vi "WILT Step Pause Dryer.vi"(7 "Station Number in":u32, 8 "Error In":errorcluster, 10 "Step 3 Input":T1, 11 "Dryer Step Pause In":T3 {"Night Cycle Count" format="%04d"; "Day Cycle Count" format="%04d"}) -> (0 "Error Out":errorcluster, 2 "Step 5 Output":T1, 3 "Dryer Step Pause Output":T3 {"Night Cycle Count" format="%04d"; "Day Cycle Count" format="%04d"})   [LabVIEW 2016]
uses:
  Type Definitions/WILT Station Test State Cluster.ctl
  Type Definitions/WILT Dryer Test State.ctl
  Type Definitions/WILT Dryer.ctl
  Type Definitions/WILT Dryer Details.ctl
  Type Definitions/WILT Agilent Channel Definition.ctl
  Type Definitions/WILT DAQ Data.ctl
  Globals/WILT Globals Main Program.vi
panel:
  # "Day"
  # "Night"
  # "Day"
  # "Night"
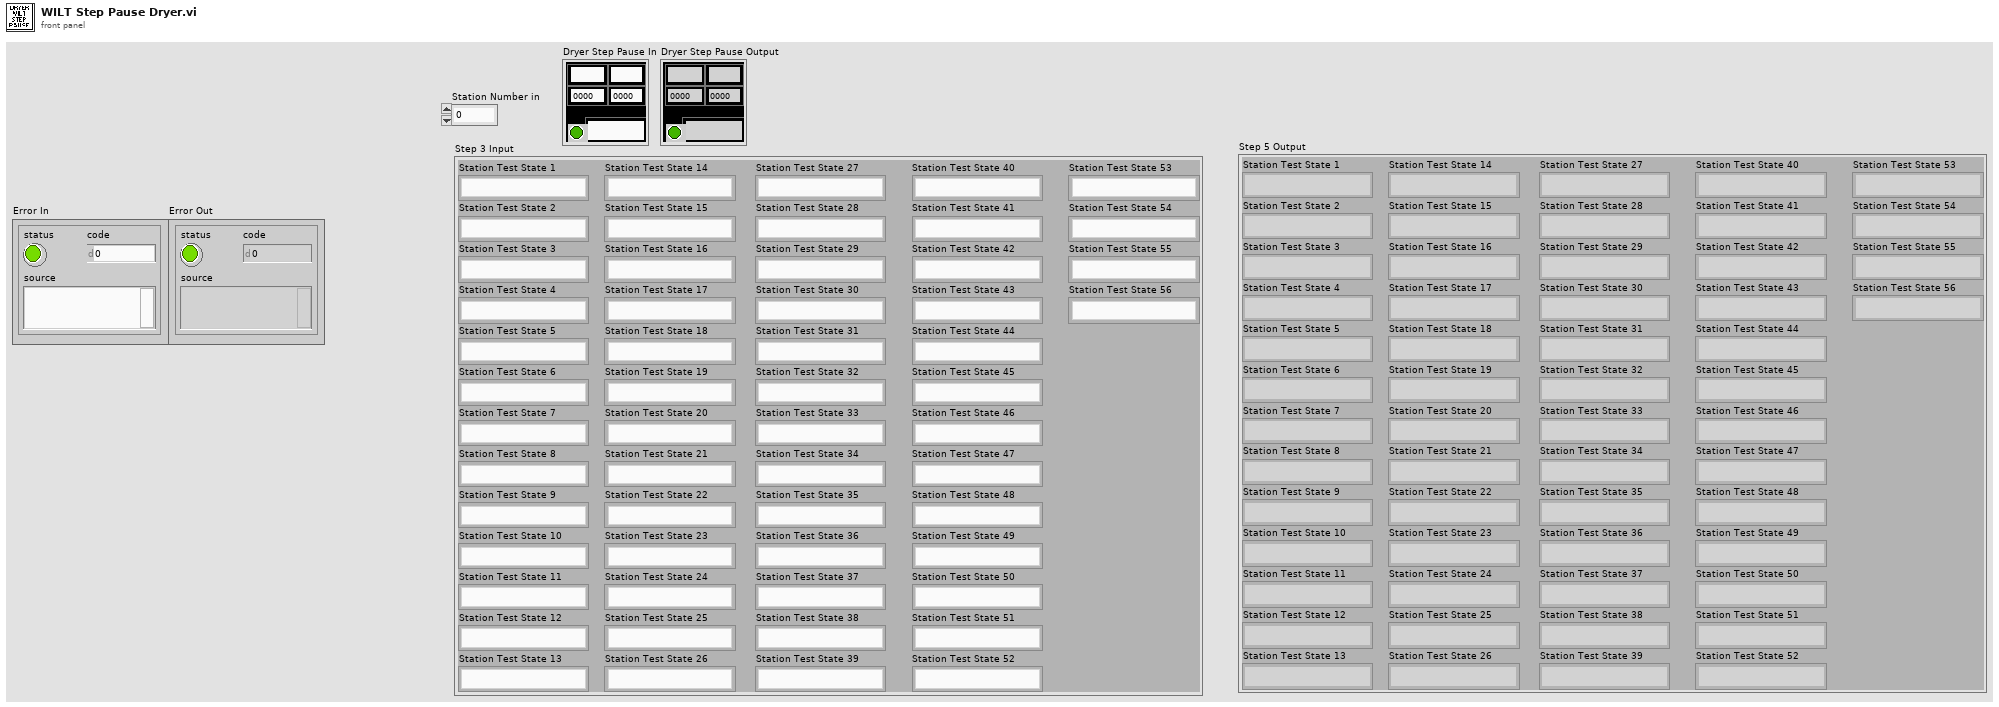
[diagram p1: front panel]
types:
  T1 = typedef "WILT Station Test State Cluster.ctl" = cluster{"Station Test State 1":T2, "Station Test State 2":T2, "Station Test State 3":T2, "Station Test State 4":T2, "Station Test State 5":T2, "Station Test State 6":T2, "Station Test State 7":T2, "Station Test State 8":T2, "Station Test State 9":T2, "Station Test State 10":T2, "Station Test State 11":T2, "Station Test State 12":T2, "Station Test State 13":T2, "Station Test State 14":T2, "Station Test State 15":T2, "Station Test State 16":T2, "Station Test State 17":T2, "Station Test State 18":T2, "Station Test State 19":T2, "Station Test State 20":T2, "Station Test State 21":T2, "Station Test State 22":T2, "Station Test State 23":T2, "Station Test State 24":T2, "Station Test State 25":T2, "Station Test State 26":T2, "Station Test State 27":T2, "Station Test State 28":T2, "Station Test State 29":T2, "Station Test State 30":T2, "Station Test State 31":T2, "Station Test State 32":T2, "Station Test State 33":T2, "Station Test State 34":T2, "Station Test State 35":T2, "Station Test State 36":T2, "Station Test State 37":T2, "Station Test State 38":T2, "Station Test State 39":T2, "Station Test State 40":T2, "Station Test State 41":T2, "Station Test State 42":T2, "Station Test State 43":T2, "Station Test State 44":T2, "Station Test State 45":T2, "Station Test State 46":T2, "Station Test State 47":T2, "Station Test State 48":T2, "Station Test State 49":T2, "Station Test State 50":T2, "Station Test State 51":T2, "Station Test State 52":T2, "Station Test State 53":T2, "Station Test State 54":T2, "Station Test State 55":T2, "Station Test State 56":T2}
  T2 = typedef "WILT Dryer Test State.ctl" = enum16{"No Serial Number", "Waiting for Dryer To Start", "Drying Clothes", "Water Injection 1 (On)", "Water Injection 1 Timer", "Water Injection 1 (Off)", "Pause Dryer", "Sending Start Stop CMD", "Pause Dryer 2", "Sending Start Stop CMD 2", "Drying Clothes 2", "Water Injection 2 (On)", "Water Injection 2 Timer", "Water Injection 2 (Off)", "Drying Clothes 3", "Cooling Down", "Sending Start Stop CMD 3", "Increment Cycle"}
  T3 = typedef "WILT Dryer.ctl" = cluster{"Lab ID":string, "Day Cycle Count":i32, "Station Label":string, "Dryer Details":T4, "Status Color":u32, "Invisible Button":bool, "Night Cycle Count":i32, "Station Index":i32, "Cycle Index":string, "Audit Alert":bool, "Agilent Channel Definition":T5, "DAQ Data":T6}
  T4 = typedef "WILT Dryer Details.ctl" = cluster{"Station":string, "Lab ID":string, "TR Number":string}
  T5 = typedef "WILT Agilent Channel Definition.ctl" = cluster{"Channel":string, "Station":string, "Label":string, "Agilent Station":string, "Data":dbl}
  T6 = typedef "WILT DAQ Data.ctl" = cluster{"L1 Current":dbl, "L2 Current":dbl, "Temperature  Deg F (TC)":dbl, "Volts":dbl, "Volts (208)":dbl, "SW (208)":dbl}
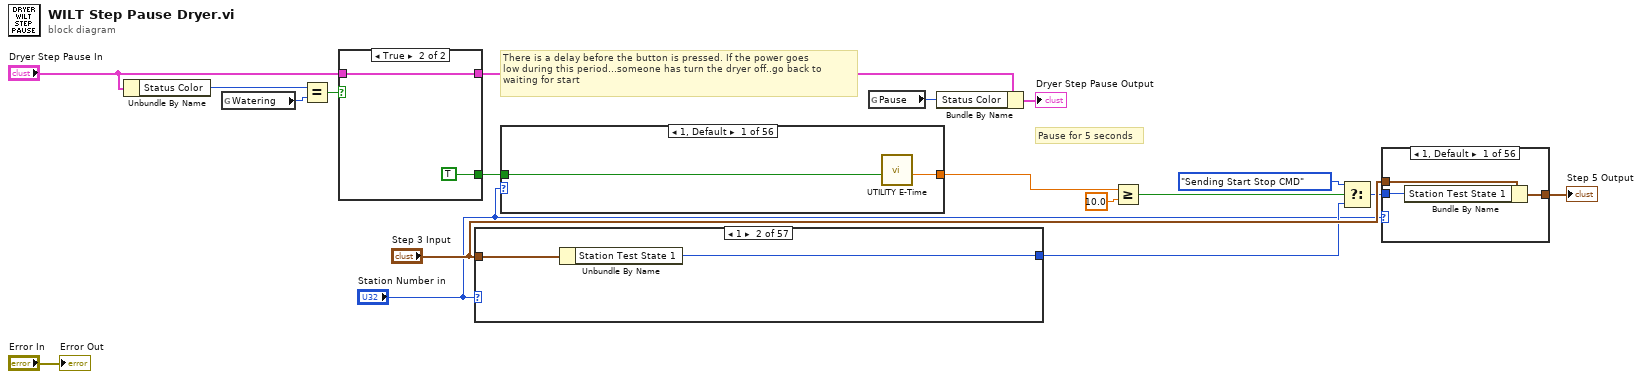
[diagram p0: block diagram]
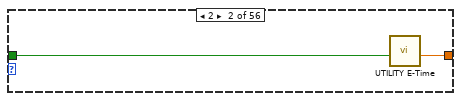
[diagram p2: hidden frame]
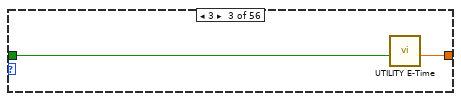
[diagram p3: hidden frame]
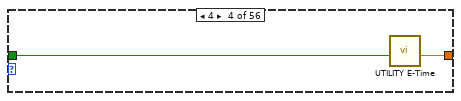
[diagram p4: hidden frame]
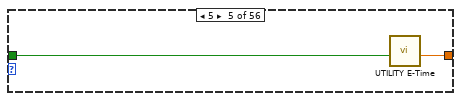
[diagram p5: hidden frame]
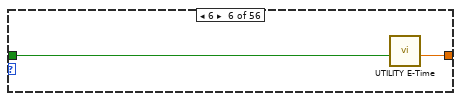
[diagram p6: hidden frame]
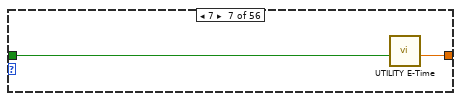
[diagram p7: hidden frame]
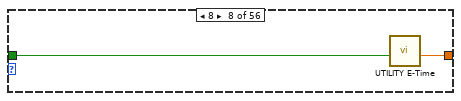
[diagram p8: hidden frame]
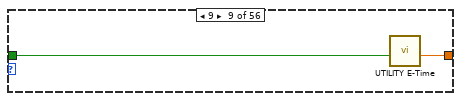
[diagram p9: hidden frame]
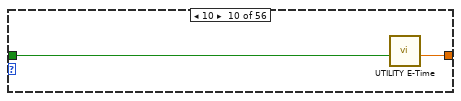
[diagram p10: hidden frame]
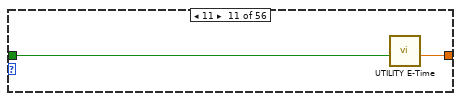
[diagram p11: hidden frame]
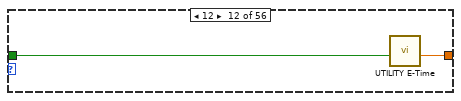
[diagram p12: hidden frame]
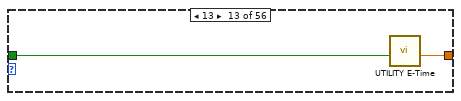
[diagram p13: hidden frame]
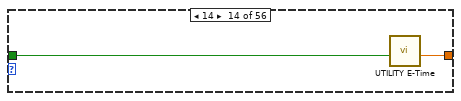
[diagram p14: hidden frame]
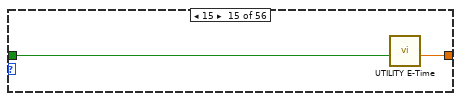
[diagram p15: hidden frame]
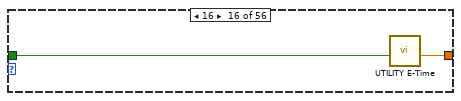
[diagram p16: hidden frame]
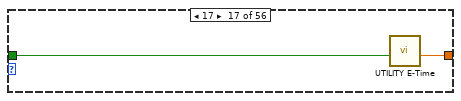
[diagram p17: hidden frame]
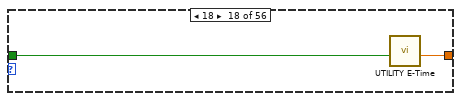
[diagram p18: hidden frame]
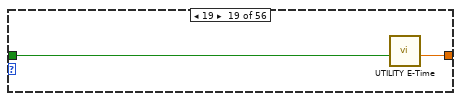
[diagram p19: hidden frame]
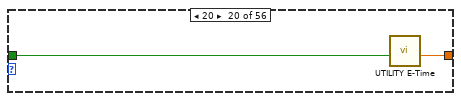
[diagram p20: hidden frame]
diagram:
  # "Pause for 5 seconds"
  # "There is a delay before the button is pressed. If the power goes\nlow during this period...someone has turn the dryer off..go back to \nwaiting for start"
  n1 = Unbundle By Name("Dryer Step Pause In") -> ("Status Color"=w12:u32)
  n2 = global read "WILT Globals Main Program.vi" "Watering"() -> (w4:u32)
  n3 = Equal?(x=w12, y=w4) -> (x = y?=w5:bool)
  n4 = case shown="True" w5 {
    tunnel: [FALSE TRUE] -> w3
    tunnel: "Dryer Step Pause In" -> [w19 w21]
    tunnel: [w19 w21] -> w2
    frame False {
    }
    frame True {
    }
  }
  n5 = case shown="1" "Station Number in" {
    tunnel: "Step 3 Input" -> [_ w25 w27 w29 w31 w33 w35 w37 w39 w41 w43 w45 w47 w49 w51 w53 w55 w57 w59 w61 w63 w65 w67 w69 w71 w73 w75 w77 w79 w81 w83 w85 w87 w89 w91 w93 w95 w97 w99 w101 w103 w105 w107 w109 w111 w113 w115 w117 w119 w121 w123 w125 w127 w129 w131 w133 w135]
    tunnel: [WILT_Dryer_Test_State."No Serial Number" ("Station Test State 56") w24 w26 w28 w30 w32 w34 w36 w38 w40 w42 w44 w46 w48 w50 w52 w54 w56 w58 w60 w62 w64 w66 w68 w70 w72 w74 w76 w78 w80 w82 w84 w86 w88 w90 w92 w94 w96 w98 w100 w102 w104 w106 w108 w110 w112 w114 w116 w118 w120 w122 w124 w126 w128 w130 w132 w134] -> w14
    frame 0, Default {
      # "This is not a station.\nDo nothing"
    }
    frame 1 {
      n6 = Unbundle By Name(w25) -> ("Station Test State 1"=w24:T2)
    }
    frame 2 {
      n7 = Unbundle By Name(w27) -> ("Station Test State 2"=w26:T2)
    }
    frame 3 {
      n8 = Unbundle By Name(w29) -> ("Station Test State 3"=w28:T2)
    }
    frame 4 {
      n9 = Unbundle By Name(w31) -> ("Station Test State 4"=w30:T2)
    }
    frame 5 {
      n10 = Unbundle By Name(w33) -> ("Station Test State 5"=w32:T2)
    }
    frame 6 {
      n11 = Unbundle By Name(w35) -> ("Station Test State 6"=w34:T2)
    }
    frame 7 {
      n12 = Unbundle By Name(w37) -> ("Station Test State 7"=w36:T2)
    }
    frame 8 {
      n13 = Unbundle By Name(w39) -> ("Station Test State 8"=w38:T2)
    }
    frame 9 {
      n14 = Unbundle By Name(w41) -> ("Station Test State 9"=w40:T2)
    }
    frame 10 {
      n15 = Unbundle By Name(w43) -> ("Station Test State 10"=w42:T2)
    }
    frame 11 {
      n16 = Unbundle By Name(w45) -> ("Station Test State 11"=w44:T2)
    }
    frame 12 {
      n17 = Unbundle By Name(w47) -> ("Station Test State 12"=w46:T2)
    }
    frame 13 {
      n18 = Unbundle By Name(w49) -> ("Station Test State 13"=w48:T2)
    }
    frame 14 {
      n19 = Unbundle By Name(w51) -> ("Station Test State 14"=w50:T2)
    }
    frame 15 {
      n20 = Unbundle By Name(w53) -> ("Station Test State 15"=w52:T2)
    }
    frame 16 {
      n21 = Unbundle By Name(w55) -> ("Station Test State 16"=w54:T2)
    }
    frame 17 {
      n22 = Unbundle By Name(w57) -> ("Station Test State 17"=w56:T2)
    }
    frame 18 {
      n23 = Unbundle By Name(w59) -> ("Station Test State 18"=w58:T2)
    }
    frame 19 {
      n24 = Unbundle By Name(w61) -> ("Station Test State 19"=w60:T2)
    }
    frame 20 {
      n25 = Unbundle By Name(w63) -> ("Station Test State 20"=w62:T2)
    }
    frame 21 {
      n26 = Unbundle By Name(w65) -> ("Station Test State 21"=w64:T2)
    }
    frame 22 {
      n27 = Unbundle By Name(w67) -> ("Station Test State 22"=w66:T2)
    }
    frame 23 {
      n28 = Unbundle By Name(w69) -> ("Station Test State 23"=w68:T2)
    }
    frame 24 {
      n29 = Unbundle By Name(w71) -> ("Station Test State 24"=w70:T2)
    }
    frame 25 {
      n30 = Unbundle By Name(w73) -> ("Station Test State 25"=w72:T2)
    }
    frame 26 {
      n31 = Unbundle By Name(w75) -> ("Station Test State 26"=w74:T2)
    }
    frame 27 {
      n32 = Unbundle By Name(w77) -> ("Station Test State 27"=w76:T2)
    }
    frame 28 {
      n33 = Unbundle By Name(w79) -> ("Station Test State 28"=w78:T2)
    }
    frame 29 {
      n34 = Unbundle By Name(w81) -> ("Station Test State 29"=w80:T2)
    }
    frame 30 {
      n35 = Unbundle By Name(w83) -> ("Station Test State 30"=w82:T2)
    }
    frame 31 {
      n36 = Unbundle By Name(w85) -> ("Station Test State 31"=w84:T2)
    }
    frame 32 {
      n37 = Unbundle By Name(w87) -> ("Station Test State 32"=w86:T2)
    }
    frame 33 {
      n38 = Unbundle By Name(w89) -> ("Station Test State 33"=w88:T2)
    }
    frame 34 {
      n39 = Unbundle By Name(w91) -> ("Station Test State 34"=w90:T2)
    }
    frame 35 {
      n40 = Unbundle By Name(w93) -> ("Station Test State 35"=w92:T2)
    }
    frame 36 {
      n41 = Unbundle By Name(w95) -> ("Station Test State 36"=w94:T2)
    }
    frame 37 {
      n42 = Unbundle By Name(w97) -> ("Station Test State 37"=w96:T2)
    }
    frame 38 {
      n43 = Unbundle By Name(w99) -> ("Station Test State 38"=w98:T2)
    }
    frame 39 {
      n44 = Unbundle By Name(w101) -> ("Station Test State 39"=w100:T2)
    }
    frame 40 {
      n45 = Unbundle By Name(w103) -> ("Station Test State 40"=w102:T2)
    }
    frame 41 {
      n46 = Unbundle By Name(w105) -> ("Station Test State 41"=w104:T2)
    }
    frame 42 {
      n47 = Unbundle By Name(w107) -> ("Station Test State 42"=w106:T2)
    }
    frame 43 {
      n48 = Unbundle By Name(w109) -> ("Station Test State 43"=w108:T2)
    }
    frame 44 {
      n49 = Unbundle By Name(w111) -> ("Station Test State 44"=w110:T2)
    }
    frame 45 {
      n50 = Unbundle By Name(w113) -> ("Station Test State 45"=w112:T2)
    }
    frame 46 {
      n51 = Unbundle By Name(w115) -> ("Station Test State 46"=w114:T2)
    }
    frame 47 {
      n52 = Unbundle By Name(w117) -> ("Station Test State 47"=w116:T2)
    }
    frame 48 {
      n53 = Unbundle By Name(w119) -> ("Station Test State 48"=w118:T2)
    }
    frame 49 {
      n54 = Unbundle By Name(w121) -> ("Station Test State 49"=w120:T2)
    }
    frame 50 {
      n55 = Unbundle By Name(w123) -> ("Station Test State 50"=w122:T2)
    }
    frame 51 {
      n56 = Unbundle By Name(w125) -> ("Station Test State 51"=w124:T2)
    }
    frame 52 {
      n57 = Unbundle By Name(w127) -> ("Station Test State 52"=w126:T2)
    }
    frame 53 {
      n58 = Unbundle By Name(w129) -> ("Station Test State 53"=w128:T2)
    }
    frame 54 {
      n59 = Unbundle By Name(w131) -> ("Station Test State 54"=w130:T2)
    }
    frame 55 {
      n60 = Unbundle By Name(w133) -> ("Station Test State 55"=w132:T2)
    }
    frame 56 {
      n61 = Unbundle By Name(w135) -> ("Station Test State 56"=w134:T2)
    }
  }
  n62 = case shown="1, Default" "Station Number in" {
    tunnel: [w137 w138 w140 w142 w144 w146 w148 w150 w152 w154 w156 w158 w160 w162 w164 w166 w168 w170 w172 w174 w176 w178 w180 w182 w184 w186 w188 w190 w192 w194 w196 w198 w200 w202 w204 w206 w208 w210 w212 w214 w216 w218 w220 w222 w224 w226 w228 w230 w232 w234 w236 w238 w240 w242 w244 w246] -> w1
    tunnel: w3 -> [w136 w139 w141 w143 w145 w147 w149 w151 w153 w155 w157 w159 w161 w163 w165 w167 w169 w171 w173 w175 w177 w179 w181 w183 w185 w187 w189 w191 w193 w195 w197 w199 w201 w203 w205 w207 w209 w211 w213 w215 w217 w219 w221 w223 w225 w227 w229 w231 w233 w235 w237 w239 w241 w243 w245 w247]
    frame 1, Default {
      n63 = call "UTILITY E-Time.vi"("Reset"=w136) -> ("Elapsed Time (sec)"=w137:dbl)  [unwired: 8 in, 2 out]
    }
    frame 2 {
      n64 = call "UTILITY E-Time.vi"("Reset"=w139) -> ("Elapsed Time (sec)"=w138:dbl)  [unwired: 8 in, 2 out]
    }
    frame 3 {
      n65 = call "UTILITY E-Time.vi"("Reset"=w141) -> ("Elapsed Time (sec)"=w140:dbl)  [unwired: 8 in, 2 out]
    }
    frame 4 {
      n66 = call "UTILITY E-Time.vi"("Reset"=w143) -> ("Elapsed Time (sec)"=w142:dbl)  [unwired: 8 in, 2 out]
    }
    frame 5 {
      n67 = call "UTILITY E-Time.vi"("Reset"=w145) -> ("Elapsed Time (sec)"=w144:dbl)  [unwired: 8 in, 2 out]
    }
    frame 6 {
      n68 = call "UTILITY E-Time.vi"("Reset"=w147) -> ("Elapsed Time (sec)"=w146:dbl)  [unwired: 8 in, 2 out]
    }
    frame 7 {
      n69 = call "UTILITY E-Time.vi"("Reset"=w149) -> ("Elapsed Time (sec)"=w148:dbl)  [unwired: 8 in, 2 out]
    }
    frame 8 {
      n70 = call "UTILITY E-Time.vi"("Reset"=w151) -> ("Elapsed Time (sec)"=w150:dbl)  [unwired: 8 in, 2 out]
    }
    frame 9 {
      n71 = call "UTILITY E-Time.vi"("Reset"=w153) -> ("Elapsed Time (sec)"=w152:dbl)  [unwired: 8 in, 2 out]
    }
    frame 10 {
      n72 = call "UTILITY E-Time.vi"("Reset"=w155) -> ("Elapsed Time (sec)"=w154:dbl)  [unwired: 8 in, 2 out]
    }
    frame 11 {
      n73 = call "UTILITY E-Time.vi"("Reset"=w157) -> ("Elapsed Time (sec)"=w156:dbl)  [unwired: 8 in, 2 out]
    }
    frame 12 {
      n74 = call "UTILITY E-Time.vi"("Reset"=w159) -> ("Elapsed Time (sec)"=w158:dbl)  [unwired: 8 in, 2 out]
    }
    frame 13 {
      n75 = call "UTILITY E-Time.vi"("Reset"=w161) -> ("Elapsed Time (sec)"=w160:dbl)  [unwired: 8 in, 2 out]
    }
    frame 14 {
      n76 = call "UTILITY E-Time.vi"("Reset"=w163) -> ("Elapsed Time (sec)"=w162:dbl)  [unwired: 8 in, 2 out]
    }
    frame 15 {
      n77 = call "UTILITY E-Time.vi"("Reset"=w165) -> ("Elapsed Time (sec)"=w164:dbl)  [unwired: 8 in, 2 out]
    }
    frame 16 {
      n78 = call "UTILITY E-Time.vi"("Reset"=w167) -> ("Elapsed Time (sec)"=w166:dbl)  [unwired: 8 in, 2 out]
    }
    frame 17 {
      n79 = call "UTILITY E-Time.vi"("Reset"=w169) -> ("Elapsed Time (sec)"=w168:dbl)  [unwired: 8 in, 2 out]
    }
    frame 18 {
      n80 = call "UTILITY E-Time.vi"("Reset"=w171) -> ("Elapsed Time (sec)"=w170:dbl)  [unwired: 8 in, 2 out]
    }
    frame 19 {
      n81 = call "UTILITY E-Time.vi"("Reset"=w173) -> ("Elapsed Time (sec)"=w172:dbl)  [unwired: 8 in, 2 out]
    }
    frame 20 {
      n82 = call "UTILITY E-Time.vi"("Reset"=w175) -> ("Elapsed Time (sec)"=w174:dbl)  [unwired: 8 in, 2 out]
    }
    frame 21 {
      n83 = call "UTILITY E-Time.vi"("Reset"=w177) -> ("Elapsed Time (sec)"=w176:dbl)  [unwired: 8 in, 2 out]
    }
    frame 22 {
      n84 = call "UTILITY E-Time.vi"("Reset"=w179) -> ("Elapsed Time (sec)"=w178:dbl)  [unwired: 8 in, 2 out]
    }
    frame 23 {
      n85 = call "UTILITY E-Time.vi"("Reset"=w181) -> ("Elapsed Time (sec)"=w180:dbl)  [unwired: 8 in, 2 out]
    }
    frame 24 {
      n86 = call "UTILITY E-Time.vi"("Reset"=w183) -> ("Elapsed Time (sec)"=w182:dbl)  [unwired: 8 in, 2 out]
    }
    frame 25 {
      n87 = call "UTILITY E-Time.vi"("Reset"=w185) -> ("Elapsed Time (sec)"=w184:dbl)  [unwired: 8 in, 2 out]
    }
    frame 26 {
      n88 = call "UTILITY E-Time.vi"("Reset"=w187) -> ("Elapsed Time (sec)"=w186:dbl)  [unwired: 8 in, 2 out]
    }
    frame 27 {
      n89 = call "UTILITY E-Time.vi"("Reset"=w189) -> ("Elapsed Time (sec)"=w188:dbl)  [unwired: 8 in, 2 out]
    }
    frame 28 {
      n90 = call "UTILITY E-Time.vi"("Reset"=w191) -> ("Elapsed Time (sec)"=w190:dbl)  [unwired: 8 in, 2 out]
    }
    frame 29 {
      n91 = call "UTILITY E-Time.vi"("Reset"=w193) -> ("Elapsed Time (sec)"=w192:dbl)  [unwired: 8 in, 2 out]
    }
    frame 30 {
      n92 = call "UTILITY E-Time.vi"("Reset"=w195) -> ("Elapsed Time (sec)"=w194:dbl)  [unwired: 8 in, 2 out]
    }
    frame 31 {
      n93 = call "UTILITY E-Time.vi"("Reset"=w197) -> ("Elapsed Time (sec)"=w196:dbl)  [unwired: 8 in, 2 out]
    }
    frame 32 {
      n94 = call "UTILITY E-Time.vi"("Reset"=w199) -> ("Elapsed Time (sec)"=w198:dbl)  [unwired: 8 in, 2 out]
    }
    frame 33 {
      n95 = call "UTILITY E-Time.vi"("Reset"=w201) -> ("Elapsed Time (sec)"=w200:dbl)  [unwired: 8 in, 2 out]
    }
    frame 34 {
      n96 = call "UTILITY E-Time.vi"("Reset"=w203) -> ("Elapsed Time (sec)"=w202:dbl)  [unwired: 8 in, 2 out]
    }
    frame 35 {
      n97 = call "UTILITY E-Time.vi"("Reset"=w205) -> ("Elapsed Time (sec)"=w204:dbl)  [unwired: 8 in, 2 out]
    }
    frame 36 {
      n98 = call "UTILITY E-Time.vi"("Reset"=w207) -> ("Elapsed Time (sec)"=w206:dbl)  [unwired: 8 in, 2 out]
    }
    frame 37 {
      n99 = call "UTILITY E-Time.vi"("Reset"=w209) -> ("Elapsed Time (sec)"=w208:dbl)  [unwired: 8 in, 2 out]
    }
    frame 38 {
      n100 = call "UTILITY E-Time.vi"("Reset"=w211) -> ("Elapsed Time (sec)"=w210:dbl)  [unwired: 8 in, 2 out]
    }
    frame 39 {
      n101 = call "UTILITY E-Time.vi"("Reset"=w213) -> ("Elapsed Time (sec)"=w212:dbl)  [unwired: 8 in, 2 out]
    }
    frame 40 {
      n102 = call "UTILITY E-Time.vi"("Reset"=w215) -> ("Elapsed Time (sec)"=w214:dbl)  [unwired: 8 in, 2 out]
    }
    frame 41 {
      n103 = call "UTILITY E-Time.vi"("Reset"=w217) -> ("Elapsed Time (sec)"=w216:dbl)  [unwired: 8 in, 2 out]
    }
    frame 42 {
      n104 = call "UTILITY E-Time.vi"("Reset"=w219) -> ("Elapsed Time (sec)"=w218:dbl)  [unwired: 8 in, 2 out]
    }
    frame 43 {
      n105 = call "UTILITY E-Time.vi"("Reset"=w221) -> ("Elapsed Time (sec)"=w220:dbl)  [unwired: 8 in, 2 out]
    }
    frame 44 {
      n106 = call "UTILITY E-Time.vi"("Reset"=w223) -> ("Elapsed Time (sec)"=w222:dbl)  [unwired: 8 in, 2 out]
    }
    frame 45 {
      n107 = call "UTILITY E-Time.vi"("Reset"=w225) -> ("Elapsed Time (sec)"=w224:dbl)  [unwired: 8 in, 2 out]
    }
    frame 46 {
      n108 = call "UTILITY E-Time.vi"("Reset"=w227) -> ("Elapsed Time (sec)"=w226:dbl)  [unwired: 8 in, 2 out]
    }
    frame 47 {
      n109 = call "UTILITY E-Time.vi"("Reset"=w229) -> ("Elapsed Time (sec)"=w228:dbl)  [unwired: 8 in, 2 out]
    }
    frame 48 {
      n110 = call "UTILITY E-Time.vi"("Reset"=w231) -> ("Elapsed Time (sec)"=w230:dbl)  [unwired: 8 in, 2 out]
    }
    frame 49 {
      n111 = call "UTILITY E-Time.vi"("Reset"=w233) -> ("Elapsed Time (sec)"=w232:dbl)  [unwired: 8 in, 2 out]
    }
    frame 50 {
      n112 = call "UTILITY E-Time.vi"("Reset"=w235) -> ("Elapsed Time (sec)"=w234:dbl)  [unwired: 8 in, 2 out]
    }
    frame 51 {
      n113 = call "UTILITY E-Time.vi"("Reset"=w237) -> ("Elapsed Time (sec)"=w236:dbl)  [unwired: 8 in, 2 out]
    }
    frame 52 {
      n114 = call "UTILITY E-Time.vi"("Reset"=w239) -> ("Elapsed Time (sec)"=w238:dbl)  [unwired: 8 in, 2 out]
    }
    frame 53 {
      n115 = call "UTILITY E-Time.vi"("Reset"=w241) -> ("Elapsed Time (sec)"=w240:dbl)  [unwired: 8 in, 2 out]
    }
    frame 54 {
      n116 = call "UTILITY E-Time.vi"("Reset"=w243) -> ("Elapsed Time (sec)"=w242:dbl)  [unwired: 8 in, 2 out]
    }
    frame 55 {
      n117 = call "UTILITY E-Time.vi"("Reset"=w245) -> ("Elapsed Time (sec)"=w244:dbl)  [unwired: 8 in, 2 out]
    }
    frame 56 {
      n118 = call "UTILITY E-Time.vi"("Reset"=w247) -> ("Elapsed Time (sec)"=w246:dbl)  [unwired: 8 in, 2 out]
    }
  }
  n119 = global read "WILT Globals Main Program.vi" "Pause"() -> (w6:u32)
  n120 = Bundle By Name(cluster=w2, "Status Color"=w6) -> (→"Dryer Step Pause Output":T3)
  n121 = Greater Or Equal?(x=w1, y=10.0) -> (x >= y?=w17:bool)
  n122 = Select(t=WILT_Dryer_Test_State."Sending Start Stop CMD" ("Current State 2"), s=w17, f=w14) -> (s? t:f=w13:T2)
  n123 = case shown="1, Default" "Station Number in" {
    tunnel: "Step 3 Input" -> [w250 w253 w256 w259 w262 w265 w268 w271 w274 w277 w280 w283 w286 w289 w292 w295 w298 w301 w304 w307 w310 w313 w316 w319 w322 w325 w328 w331 w334 w337 w340 w343 w346 w349 w352 w355 w358 w361 w364 w367 w370 w373 w376 w379 w382 w385 w388 w391 w394 w397 w400 w403 w406 w409 w412 w415]
    tunnel: w13 -> [w249 w251 w254 w257 w260 w263 w266 w269 w272 w275 w278 w281 w284 w287 w290 w293 w296 w299 w302 w305 w308 w311 w314 w317 w320 w323 w326 w329 w332 w335 w338 w341 w344 w347 w350 w353 w356 w359 w362 w365 w368 w371 w374 w377 w380 w383 w386 w389 w392 w395 w398 w401 w404 w407 w410 w413]
    tunnel: [w248 w252 w255 w258 w261 w264 w267 w270 w273 w276 w279 w282 w285 w288 w291 w294 w297 w300 w303 w306 w309 w312 w315 w318 w321 w324 w327 w330 w333 w336 w339 w342 w345 w348 w351 w354 w357 w360 w363 w366 w369 w372 w375 w378 w381 w384 w387 w390 w393 w396 w399 w402 w405 w408 w411 w414] -> w16
    frame 1, Default {
      n124 = Bundle By Name(cluster=w250, "Station Test State 1"=w249) -> (w248:T1)
    }
    frame 2 {
      n125 = Bundle By Name(cluster=w253, "Station Test State 2"=w251) -> (w252:T1)
    }
    frame 3 {
      n126 = Bundle By Name(cluster=w256, "Station Test State 3"=w254) -> (w255:T1)
    }
    frame 4 {
      n127 = Bundle By Name(cluster=w259, "Station Test State 4"=w257) -> (w258:T1)
    }
    frame 5 {
      n128 = Bundle By Name(cluster=w262, "Station Test State 5"=w260) -> (w261:T1)
    }
    frame 6 {
      n129 = Bundle By Name(cluster=w265, "Station Test State 6"=w263) -> (w264:T1)
    }
    frame 7 {
      n130 = Bundle By Name(cluster=w268, "Station Test State 7"=w266) -> (w267:T1)
    }
    frame 8 {
      n131 = Bundle By Name(cluster=w271, "Station Test State 8"=w269) -> (w270:T1)
    }
    frame 9 {
      n132 = Bundle By Name(cluster=w274, "Station Test State 9"=w272) -> (w273:T1)
    }
    frame 10 {
      n133 = Bundle By Name(cluster=w277, "Station Test State 10"=w275) -> (w276:T1)
    }
    frame 11 {
      n134 = Bundle By Name(cluster=w280, "Station Test State 11"=w278) -> (w279:T1)
    }
    frame 12 {
      n135 = Bundle By Name(cluster=w283, "Station Test State 12"=w281) -> (w282:T1)
    }
    frame 13 {
      n136 = Bundle By Name(cluster=w286, "Station Test State 13"=w284) -> (w285:T1)
    }
    frame 14 {
      n137 = Bundle By Name(cluster=w289, "Station Test State 14"=w287) -> (w288:T1)
    }
    frame 15 {
      n138 = Bundle By Name(cluster=w292, "Station Test State 15"=w290) -> (w291:T1)
    }
    frame 16 {
      n139 = Bundle By Name(cluster=w295, "Station Test State 16"=w293) -> (w294:T1)
    }
    frame 17 {
      n140 = Bundle By Name(cluster=w298, "Station Test State 17"=w296) -> (w297:T1)
    }
    frame 18 {
      n141 = Bundle By Name(cluster=w301, "Station Test State 18"=w299) -> (w300:T1)
    }
    frame 19 {
      n142 = Bundle By Name(cluster=w304, "Station Test State 19"=w302) -> (w303:T1)
    }
    frame 20 {
      n143 = Bundle By Name(cluster=w307, "Station Test State 20"=w305) -> (w306:T1)
    }
    frame 21 {
      n144 = Bundle By Name(cluster=w310, "Station Test State 21"=w308) -> (w309:T1)
    }
    frame 22 {
      n145 = Bundle By Name(cluster=w313, "Station Test State 22"=w311) -> (w312:T1)
    }
    frame 23 {
      n146 = Bundle By Name(cluster=w316, "Station Test State 23"=w314) -> (w315:T1)
    }
    frame 24 {
      n147 = Bundle By Name(cluster=w319, "Station Test State 24"=w317) -> (w318:T1)
    }
    frame 25 {
      n148 = Bundle By Name(cluster=w322, "Station Test State 25"=w320) -> (w321:T1)
    }
    frame 26 {
      n149 = Bundle By Name(cluster=w325, "Station Test State 26"=w323) -> (w324:T1)
    }
    frame 27 {
      n150 = Bundle By Name(cluster=w328, "Station Test State 27"=w326) -> (w327:T1)
    }
    frame 28 {
      n151 = Bundle By Name(cluster=w331, "Station Test State 28"=w329) -> (w330:T1)
    }
    frame 29 {
      n152 = Bundle By Name(cluster=w334, "Station Test State 29"=w332) -> (w333:T1)
    }
    frame 30 {
      n153 = Bundle By Name(cluster=w337, "Station Test State 30"=w335) -> (w336:T1)
    }
    frame 31 {
      n154 = Bundle By Name(cluster=w340, "Station Test State 31"=w338) -> (w339:T1)
    }
    frame 32 {
      n155 = Bundle By Name(cluster=w343, "Station Test State 32"=w341) -> (w342:T1)
    }
    frame 33 {
      n156 = Bundle By Name(cluster=w346, "Station Test State 33"=w344) -> (w345:T1)
    }
    frame 34 {
      n157 = Bundle By Name(cluster=w349, "Station Test State 34"=w347) -> (w348:T1)
    }
    frame 35 {
      n158 = Bundle By Name(cluster=w352, "Station Test State 35"=w350) -> (w351:T1)
    }
    frame 36 {
      n159 = Bundle By Name(cluster=w355, "Station Test State 36"=w353) -> (w354:T1)
    }
    frame 37 {
      n160 = Bundle By Name(cluster=w358, "Station Test State 37"=w356) -> (w357:T1)
    }
    frame 38 {
      n161 = Bundle By Name(cluster=w361, "Station Test State 38"=w359) -> (w360:T1)
    }
    frame 39 {
      n162 = Bundle By Name(cluster=w364, "Station Test State 39"=w362) -> (w363:T1)
    }
    frame 40 {
      n163 = Bundle By Name(cluster=w367, "Station Test State 40"=w365) -> (w366:T1)
    }
    frame 41 {
      n164 = Bundle By Name(cluster=w370, "Station Test State 41"=w368) -> (w369:T1)
    }
    frame 42 {
      n165 = Bundle By Name(cluster=w373, "Station Test State 42"=w371) -> (w372:T1)
    }
    frame 43 {
      n166 = Bundle By Name(cluster=w376, "Station Test State 43"=w374) -> (w375:T1)
    }
    frame 44 {
      n167 = Bundle By Name(cluster=w379, "Station Test State 44"=w377) -> (w378:T1)
    }
    frame 45 {
      n168 = Bundle By Name(cluster=w382, "Station Test State 45"=w380) -> (w381:T1)
    }
    frame 46 {
      n169 = Bundle By Name(cluster=w385, "Station Test State 46"=w383) -> (w384:T1)
    }
    frame 47 {
      n170 = Bundle By Name(cluster=w388, "Station Test State 47"=w386) -> (w387:T1)
    }
    frame 48 {
      n171 = Bundle By Name(cluster=w391, "Station Test State 48"=w389) -> (w390:T1)
    }
    frame 49 {
      n172 = Bundle By Name(cluster=w394, "Station Test State 49"=w392) -> (w393:T1)
    }
    frame 50 {
      n173 = Bundle By Name(cluster=w397, "Station Test State 50"=w395) -> (w396:T1)
    }
    frame 51 {
      n174 = Bundle By Name(cluster=w400, "Station Test State 51"=w398) -> (w399:T1)
    }
    frame 52 {
      n175 = Bundle By Name(cluster=w403, "Station Test State 52"=w401) -> (w402:T1)
    }
    frame 53 {
      n176 = Bundle By Name(cluster=w406, "Station Test State 53"=w404) -> (w405:T1)
    }
    frame 54 {
      n177 = Bundle By Name(cluster=w409, "Station Test State 54"=w407) -> (w408:T1)
    }
    frame 55 {
      n178 = Bundle By Name(cluster=w412, "Station Test State 55"=w410) -> (w411:T1)
    }
    frame 56 {
      n179 = Bundle By Name(cluster=w415, "Station Test State 56"=w413) -> (w414:T1)
    }
  }
  "Step 5 Output" <- w16
  "Error Out" <- "Error In"
